vi "Set VDD Voltage and MeasV_w_Delay.vi"(0 "Semiconductor Module Context":T1, 1 "Publishable ID":string="PreFuse_Vio_Meas", 2 "Delay_after_Power_Up":dbl=0.001 format="%#_13p", 5 "Pins":string[](array[string])=["VDD"], 7 "Bridge_VSU_Supply":string="VSU", 9 "VDD voltage level":dbl=1.8 caption="voltage level" format="%_6p", 11 "error in (no error)":errorcluster) -> (4 "Semiconductor Module Context Out":T1, 6 "Instrument Sessions Out":refnum<k15>[](array[refnum]), 15 "error out":errorcluster)   [LabVIEW 2013]
uses:
  <vilib>/NI_TestStand_SemiconductorModule/NI_TestStand_Semiconductor_Module.lvlibp/PinMap/General/SemiconductorModuleContext.ctl
  <vilib>/NI_TestStand_SemiconductorModule/NI_TestStand_Semiconductor_Module.lvlibp/PinMap/DC Power/PinsToNIDCPowerSessions.vi
  <vilib>/NI_TestStand_SemiconductorModule/NI_TestStand_Semiconductor_Module.lvlibp/PinMap/Deprecated/PublishDataDoubleSinglePinSingleInstrument.vi
  <vilib>/NI_TestStand_SemiconductorModule/NI_TestStand_Semiconductor_Module.lvlibp
panel:
  out "voltage measurements":dbl[][](array[numeric])
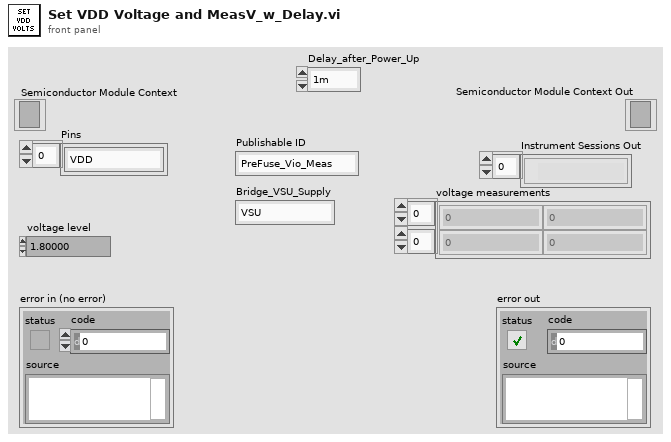
[diagram p1: front panel]
types:
  T1 = typedef "NI_TestStand_Semiconductor_Module.lvlibp/SemiconductorModuleContext.ctl" = refnum<k7>
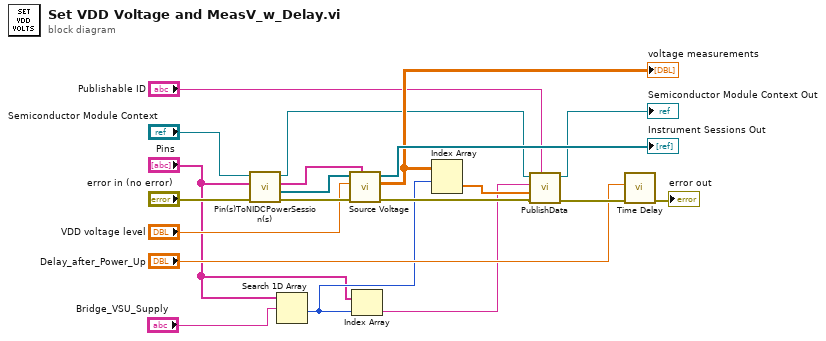
[diagram p0: block diagram]
diagram:
  n1 = call-poly <vilib>:"Pin(s)ToNIDCPowerSession(s).vi"("error in (no error)"="error in (no error)", "Pins"="Pins", "Semiconductor Module Context"="Semiconductor Module Context") -> ("error out"=w18:errorcluster, "Instrument Sessions"=w17:refnum<k15>[], "Channel Lists"=w4:string[], "Semiconductor Module Context Out"=w11:T1)  [unwired: 4 in, 1 out]
  n2 = Search 1D Array(1D array="Pins", element="Bridge_VSU_Supply") -> (index of element=w3:i32)  [unwired: 1 in]
  n3 = call "Source Voltage.vi"("Channel Lists"=w4, "error in (no error)"=w18, "voltage level"="VDD voltage level", "Instrument Sessions In"=w17) -> ("error out"=w13:errorcluster, "voltage measurements"=w14:dbl[][], "Instrument Sessions Out"=→"Instrument Sessions Out":refnum<k15>[])  [unwired: 4 in, 1 out]
  "voltage measurements" <- w14
  n4 = Index Array(array="Pins", index=w3) -> (element=w2:string)
  n5 = Index Array(array=w14, index (row)=w3) -> (element=w9:dbl[])  [unwired: 1 in]
  n6 = call-poly <vilib>:"PublishData.vi"("Measurement Id"="Publishable ID", "error in (no error)"=w13, "Data In"=w9, "Pin"=w2, "Semiconductor Module Context"=w11) -> ("error out"=w8:errorcluster, "Semiconductor Module Context Out"=→"Semiconductor Module Context Out":T1)  [unwired: 5 in]
  n7 = call "Time Delay"("error in (no error)"=w8, "Delay Time (s)"="Delay_after_Power_Up") -> ("error out"=→"error out":errorcluster)  [unwired: 9 in]
